vi "Autonomous Independent.vi"() -> ()   [LabVIEW 2015]
doc: "This VI is called when autonomous begins, and will automatically be terminated when autonomous ends. You can carry out timed or sensor driven robot movement independently without needing to return to the caller."
uses:
  Lightning/Support/LightningPID Settings.ctl
  Lightning/Auton/AutonStates.ctl
panel:
  in  "Use Ave":bool=TRUE
  in  "Kv":dbl=0.09 format="%#_13g"
  in  "Ka":dbl=0.02 format="%#_13g"
  in  "PID Settings":T1
  out "file error":errorcluster
  # "Be sure to right-click and choose Data Operations>>Make Current Value default if you want to save the array values with the VI"
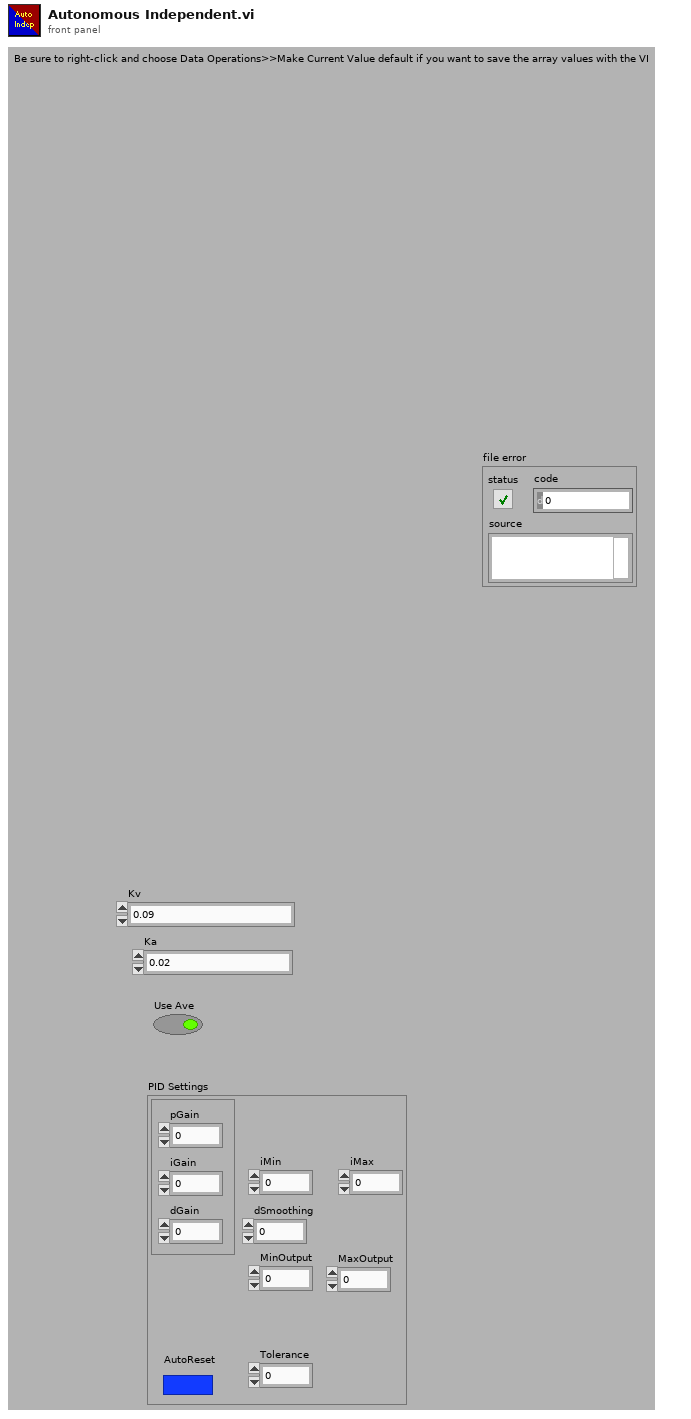
[diagram p1: front panel]
types:
  T1 = typedef "LightningPID Settings.ctl" = cluster{"iMax":dbl, "iMin":dbl, "iGain":dbl, "pGain":dbl, "dGain":dbl, "MaxOutput":dbl, "MinOutput":dbl, "AutoReset":bool, "Tolerance":dbl, "dSmoothing":dbl}
  T2 = typedef "AutonStates.ctl" = enum16{"Autobots Roll Up", "Follow Test Track", "Moat High", "Moat Low", "Rockwall High", "Rockwall Low", "Ramparts High", "Ramparts Low", "RoTe High", "Ramparts", "Rote Low"}
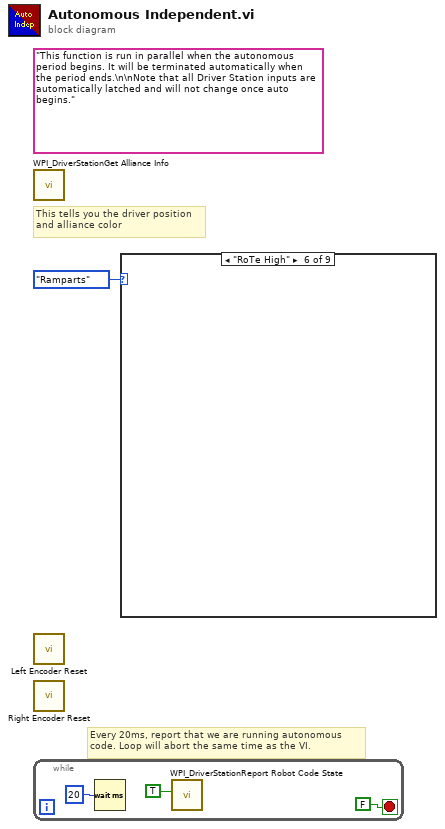
[diagram p0: block diagram]
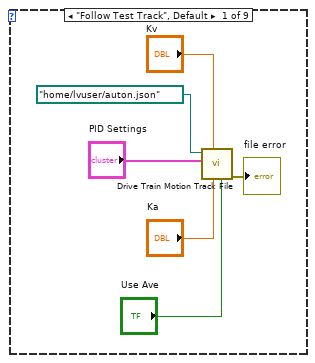
[diagram p2: hidden frame]
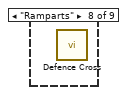
[diagram p8: hidden frame]
diagram:
  (unwired) "This function is run in parallel when the autonomous period begins. It will be terminated automatically when the period ends.\n\nNote that all Driver Station inputs are automatically latched and will not change once auto begins."
  # "Every 20ms, report that we are running autonomous\ncode. Loop will abort the same time as the VI."
  # "This tells you the driver position\nand alliance color"
  n1 = call <vilib>:"WPI_DriverStationGet Alliance Info.vi"() -> ()  [unwired: 12 out]
  n2 = call "Left Encoder Reset.vi"() -> ()  [unwired: 12 in]
  n3 = call "Right Encoder Reset.vi"() -> ()  [unwired: 12 in]
  n4 = while {
    stop <- FALSE stop-if-true
    n5 = Wait (ms)(milliseconds to wait=u32 20) -> ()  [unwired: 1 out]
    n6 = call <vilib>:"WPI_DriverStationReport Robot Code State.vi"("Autonomous"=TRUE) -> ()  [unwired: 10 in, 1 out]
  }
  n7 = case shown="\"RoTe High\"" AutonStates."Ramparts" {
    frame "Follow Test Track", Default {
      n8 = call "Drive Train Motion Track File.vi"("Use Ave"="Use Ave", "Ka"="Ka", "Kv"="Kv", "PID Settings"="PID Settings", "file (use dialog)"=path "/home/lvuser/auton.json") -> ("error out"=→"file error":errorcluster)  [unwired: 5 in, 1 out]
    }
    frame "Moat High" {
    }
    frame "Moat Low" {
    }
    frame "Rockwall High" {
    }
    frame "Rockwall Low" {
    }
    frame "RoTe High" {
    }
    frame "Rote Low" {
    }
    frame "Ramparts" {
      n9 = call "Defence Cross.vi"() -> ()  [unwired: 12 in]
    }
    frame "Autobots Roll Up" {
    }
  }
